vi "Output_Displacement.vi"() -> (5 "Plug in titles":string[](array[string]), 7 "Plug in values":string[](array[string]))   [LabVIEW 2018]
uses:
  ADAM Client/Sub VIs/ADAM Controls/Update_scan_value.ctl
  Globals/Meas_global.vi
panel:
  # "Please enter any run information in the box below"
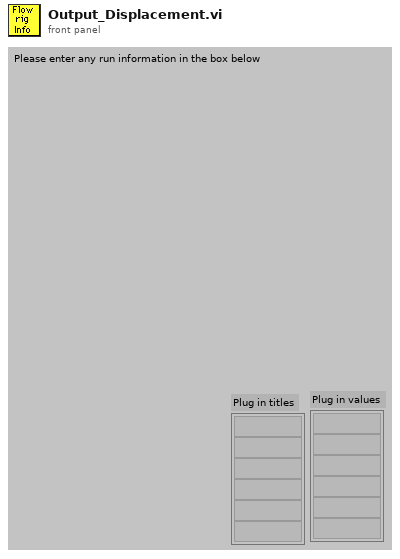
[diagram p1: front panel]
types:
  T1 = typedef "Update_scan_value.ctl" = cluster{"Channel Name":string, "New Value":dbl}
  T2 = typedef "Analysis_info_cluster.ctl" = cluster{"Colour":u32, "Inst type":T3, "Inst name":string, "Symbol":string, "Code name":string, "Extra Info":string, "Inst Array":T4, "Extra Titles":string[], "Extra Values":string[], "U":dbl, "u^2":dbl, "u^3":dbl, "u^4":dbl, "Skew_u":dbl, "Kurt_u":dbl, "Sd Error in Mean":dbl, "% u'/U":dbl, "X":dbl, "Y":dbl, "Z":dbl, "Timescale integral Estimate":dbl, "Sd Error in Variance":dbl, "Calib File":path, "Calib Constants":dbl[], "Output Position":bool, "Stats":enum16{"None", "Basic", "Full"}, "Av Sampling Rate":dbl, "Av No of Samples":dbl, "Total Meas Time (s)":dbl, "ADAM Ch Name":string, "Max value":dbl, "Min value":dbl, "Req Sample Rate Hz":dbl, "Sync Delay Time (s)":dbl, "Ch No":i16, "Device":string, "Use Latest Calib":bool, "Port":string, "Metadata Ch Names":string[], "Metadata Ch Values":string[]}
  T3 = typedef "Inst_type.ctl" = enum16{"Propeller anemometer", "Raw voltage", "Pressure Transducer", "Pitot-static tube", "Preston tube", "Hot wire", "Cross wire 1", "Cross wire 2", "Generic Linear", "Generic Polynomial", "Generic BackPoly", "Fast FID", "Thermocouple", "Cold wire", "Pulsed Wire", "LDA Vel", "LDA Tran time", "LDA Arr time", "Microphone"}
  T4 = typedef "Instrument_Array.ctl" = enum16{"PWA", "LDA", "Analogue"}
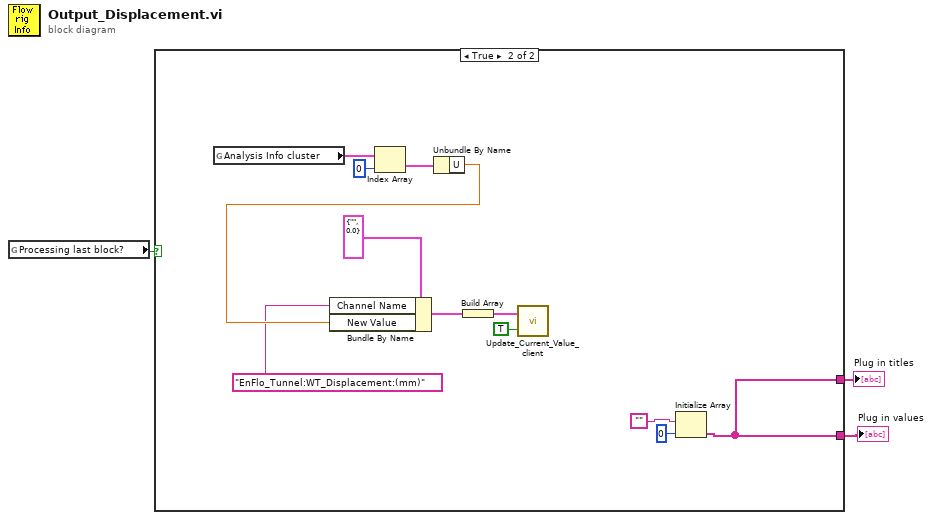
[diagram p0: block diagram]
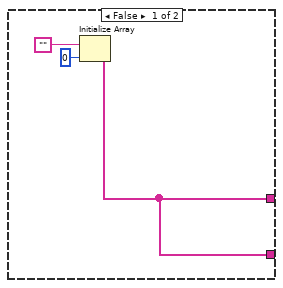
[diagram p2: hidden frame]
diagram:
  n1 = global read "Meas_global.vi" "Processing last block?"() -> (w3:bool)
  n2 = case shown="True" w3 {
    tunnel: [w4 w18] -> w2
    tunnel: [w4 w18] -> w1
    frame False {
      n3 = Initialize Array("", 0) -> (w4:string[])
    }
    frame True {
      n4 = global read "Meas_global.vi" "Analysis Info cluster"() -> (w17:T2[])
      n5 = Index Array(array=w17, index=0) -> (element=w15:T2)
      n6 = Unbundle By Name(w15) -> ("U"=w11:dbl)
      n7 = Bundle By Name(cluster=T1 {"Channel Name"="", "New Value"=0.0} ("Update Scan Value Cluster"), "Channel Name"="EnFlo_Tunnel:WT_Displacement:(mm)", "New Value"=w11) -> (w9:T1)
      n8 = Build Array(w9) -> (w8:T1[])
      n9 = call "Update_Current_Value_client.vi"("Don't Bother with check?"=TRUE, "Update array in"=w8) -> ()
      n10 = Initialize Array("", 0) -> (w18:string[])
    }
  }
  "Plug in titles" <- w2
  "Plug in values" <- w1
